vi "CheckIfTempExceed.vi"(8 "error in (no error)":errorcluster, 10 "MeasData":dbl[](array[numeric]), 11 "4118 in":refnum<class "4118.lvclass">) -> (0 "error out":errorcluster, 3 "4118 out":refnum<class "4118.lvclass">)   [LabVIEW 2024, in "4118 Actor.lvlib" / "4118.lvclass"]
uses:
  4118.lvclass
  C:/Program Files (x86)/National Instruments/LabVIEW 2024/vi.lib/ActorFramework/Actor/Actor.lvclass
  4118.lvclass/4118.ctl
  MFActor/ActorMessage/MF Task Name.ctl
  <vilib>/ActorFramework/Actor/Actor.lvclass/Actor.ctl
  <vilib>/ActorFramework/Actor/Actor.lvclass
  MFActor/ActorMessage/MFActorMsg.lvclass
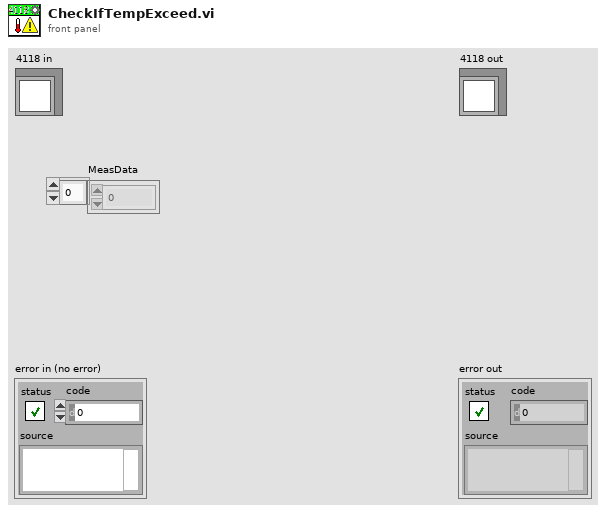
[diagram p1: front panel]
types:
  T1 = typedef "MF Task Name.ctl" = enum16{"DIChanged", "UpdateErrorCode", "SetTorque", "SetDriveTorque", "DataUpdated", "RunningTestProc", "StreamCtrl", "RunPID", "StopTest", "TCP Conn", "RefreshAutoUI", "ZeroAngle", "NestedActorLaunched", "NestedActorEnded", "ShowPsMsg"}
  T2 = cluster{"Interface":refnum<visa-resource-name>, "value range":string, "Channel Count":i32, "Limit 0":dbl, "Limit 1":dbl, "Limit 2":dbl, "Limit 3":dbl, "Limit 4":dbl, "Limit 5":dbl, "Limit 6":dbl, "Limit 7":dbl}
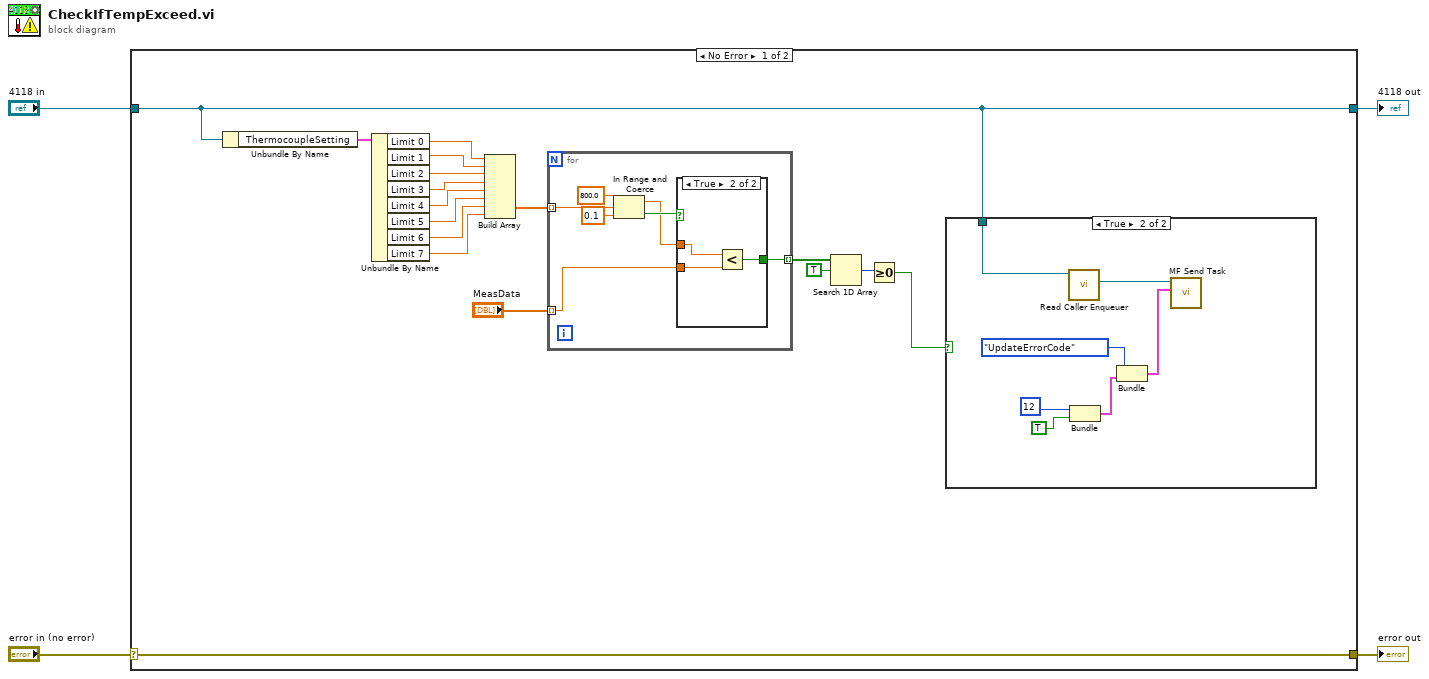
[diagram p0: block diagram]
diagram:
  n1 = case shown="No Error" "error in (no error)" {
    selector: "error in (no error)" -> [w21 w40]
    tunnel: [w21 w40] -> w3
    tunnel: [w5 w39] -> w1
    tunnel: "4118 in" -> [w5 w39]
    frame No Error {
      n2 = Unbundle By Name(w5) -> ("ThermocoupleSetting"=w20:T2)
      n3 = Unbundle By Name(w20) -> ("Limit 0"=w19:dbl, "Limit 1"=w18:dbl, "Limit 2"=w17:dbl, "Limit 3"=w16:dbl, "Limit 4"=w15:dbl, "Limit 5"=w14:dbl, "Limit 6"=w13:dbl, "Limit 7"=w12:dbl)
      n4 = Build Array(w19, w18, w17, w16, w15, w14, w13, w12) -> (w11:dbl[])
      n5 = for {
        tunnel: w11 -> [w35] mode=indexing
        tunnel: "MeasData" -> [w30] mode=indexing
        tunnel: [w29] -> w9 mode=indexing
        n6 = In Range and Coerce(upper limit=800.0, x=w35, lower limit=0.1) -> (coerced(x)=w31:dbl, In Range?=w32:bool)
        n7 = case shown="True" w32 {
          tunnel: w31 -> [_ w38]
          tunnel: w30 -> [_ w37]
          tunnel: [_ w36] -> w29
          frame False {
          }
          frame True {
            n8 = Less?(x=w38, y=w37) -> (x < y?=w36:bool)
          }
        }
      }
      n9 = Search 1D Array(1D array=w9, element=TRUE) -> (index of element=w7:i32)  [unwired: 1 in]
      n10 = Greater Or Equal To 0?(x=w7) -> (x >= 0?=w6:bool)
      n11 = case shown="True" w6 {
        tunnel: w5 -> [_ w27]
        frame False {
        }
        frame True {
          n12 = call <vilib>:"Read Caller Enqueuer.vi"("Actor"=w27) -> ("Caller Enqueuer"=w28:refnum<class "Message Enqueuer.lvclass">)  [unwired: 10 in]
          n13 = Bundle(12, TRUE) -> (w23:cluster{i32, bool})  [unwired: 1 in]
          n14 = Bundle("MF Msg Enum"=MF_Task_Name."UpdateErrorCode", w23) -> (w22:cluster{"MF Msg Enum":T1, cluster{i32, bool}})  [unwired: 1 in]
          n15 = call "MF Send Task.vi"("MsgType"=w22, "Message Enqueuer"=w28) -> ()  [unwired: 9 in, 1 out]
        }
      }
    }
    frame Error {
    }
  }
  "error out" <- w3
  "4118 out" <- w1
